vi "niScope Configure Trigger Glitch.vi"(0 "instrument handle":refnum<k15>, 1 "polarity":T2=1 items=["Positive"=1, "Negative"=2, "Either"=3], 2 "trigger coupling":T4=1 items=["AC"=0, "DC"=1, "HF Reject"=3, "LF Reject"=4, "AC Plus HF Reject"=1001], 3 "width":dbl format="%.2f", 5 "trigger source":T3="0", 7 "trigger level":dbl format="%.2f", 9 "glitch condition":T1=2 items=["Less Than"=1, "Greater Than"=2], 11 "error in":errorcluster, 12 "trigger holdoff":dbl format="%.4f", 13 "trigger delay":dbl format="%.4f") -> (4 "instrument handle out":refnum<k15>, 15 "error out":errorcluster)   [LabVIEW 2020]
doc: "Configures common properties for glitch triggering."
uses:
  niScope trigger coupling.ctl
  niScope trigger source.ctl
  niScope trigger polarity.ctl
  niScope glitch condition.ctl
  niScope_32.dll
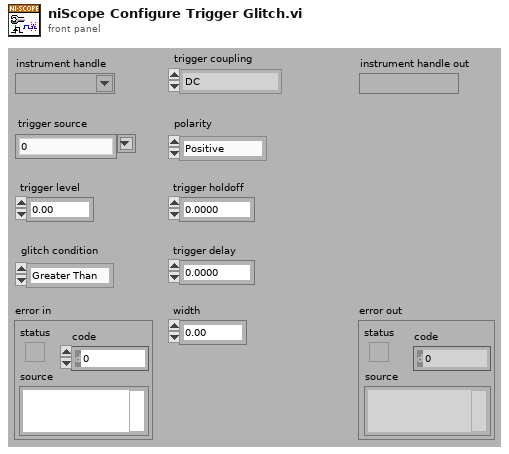
[diagram p1: front panel]
types:
  T1 = typedef "niScope glitch condition.ctl" = i32
  T2 = typedef "niScope trigger polarity.ctl" = i32
  T3 = typedef "niScope trigger source.ctl" = string
  T4 = typedef "niScope trigger coupling.ctl" = u16
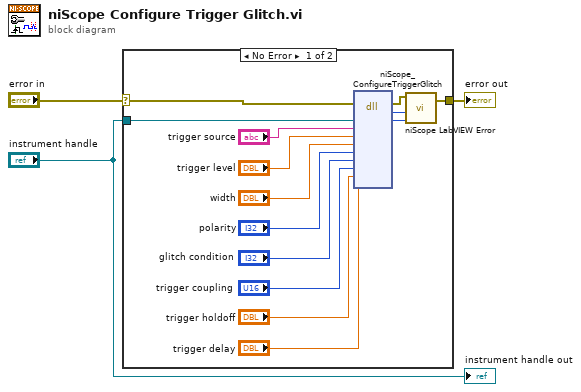
[diagram p0: block diagram]
diagram:
  n1 = case shown="No Error" "error in" {
    selector: "error in" -> [w5 w18]
    tunnel: [w14 w18] -> w3
    tunnel: "instrument handle" -> [w17 _]
    frame No Error {
      n2 = dll-call lib="niScope_*.*" fn="niScope_ConfigureTriggerGlitch"(error in=w5, "instrument handle"=w17, "triggerSource"="trigger source", "level"="trigger level", "glitchWidth"="width", "glitchPolarity"="polarity", "glitchCondition"="glitch condition", "coupling"="trigger coupling", "holdoff"="trigger holdoff", "delay"="trigger delay") -> (error out=w4:errorcluster, "status"=w16:i32, "instrument handle"=w15:u32)  [unwired: 10 in, 1 out]
      n3 = call "niScope LabVIEW Error.vi"("instrument handle"=w15, "niScope error code (0)"=w16, "error in (no error)"=w4) -> ("error out"=w14:errorcluster)  [unwired: 2 in]
    }
    frame Error {
    }
  }
  "error out" <- w3
  "instrument handle out" <- "instrument handle"
